vi "Tell.vi"(4 "Priority":bool, 10 "Msg":refnum<class "Msg.lvclass">, 11 "Transport in":refnum<class "Transport.lvclass">) -> (0 "Error out":errorcluster)   [LabVIEW 2020, in "jettl.lvlib" / "Transport.lvclass"]
uses:
  Transport.lvclass
  Msg/Msg.lvclass
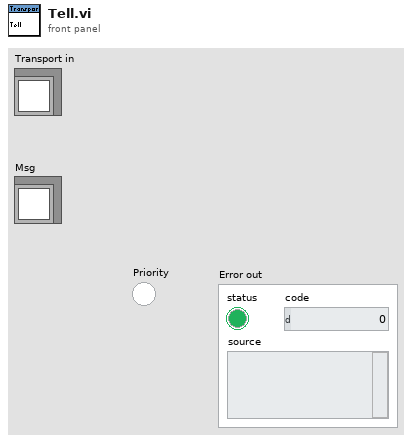
[diagram p1: front panel]
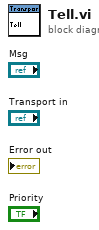
[diagram p0: block diagram]
diagram:
